vi "port_waveform_builder.vi"(4 "Line 7":digitalwaveform(waveform)={"t0"=timestamp(0 s since 1904-01-01), "dt"=0.0, "Y"={"transitions"=[], "data"=[]}, "error"={"status"=FALSE, "code"=37421928, "source"=""}}, 6 "Line 6":digitalwaveform(waveform)={"t0"=timestamp(0 s since 1904-01-01), "dt"=0.0, "Y"={"transitions"=[], "data"=[]}, "error"={"status"=FALSE, "code"=37421928, "source"=""}}, 7 "Line 1":digitalwaveform(waveform)={"t0"=timestamp(0 s since 1904-01-01), "dt"=0.0, "Y"={"transitions"=[], "data"=[]}, "error"={"status"=FALSE, "code"=37421928, "source"=""}}, 8 "Line 5":digitalwaveform(waveform)={"t0"=timestamp(0 s since 1904-01-01), "dt"=0.0, "Y"={"transitions"=[], "data"=[]}, "error"={"status"=FALSE, "code"=37421928, "source"=""}}, 11 "Line 2":digitalwaveform(waveform)={"t0"=timestamp(0 s since 1904-01-01), "dt"=0.0, "Y"={"transitions"=[], "data"=[]}, "error"={"status"=FALSE, "code"=37421928, "source"=""}}) -> (3 "digital waveform out":digitalwaveform(waveform)={"t0"=timestamp(0 s since 1904-01-01), "dt"=0.0, "Y"={"transitions"=[], "data"=[]}, "error"={"status"=FALSE, "code"=37421928, "source"=""}})   [LabVIEW 2012]
uses:
  <vilib>/Waveform/DWDTOps.llb/DWDT Append Digital Signals.vi
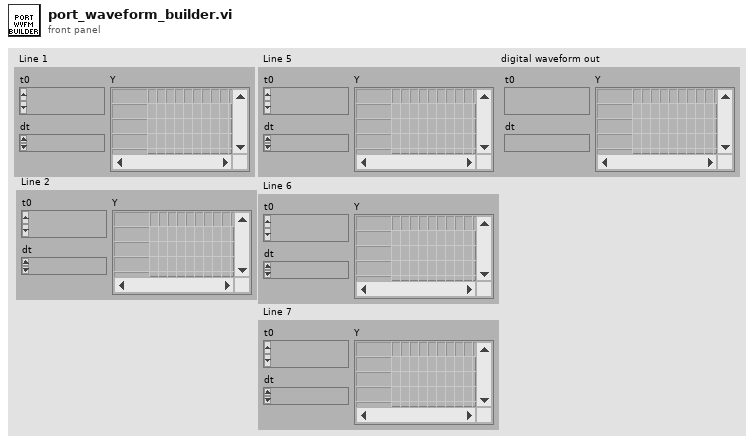
[diagram p1: front panel]
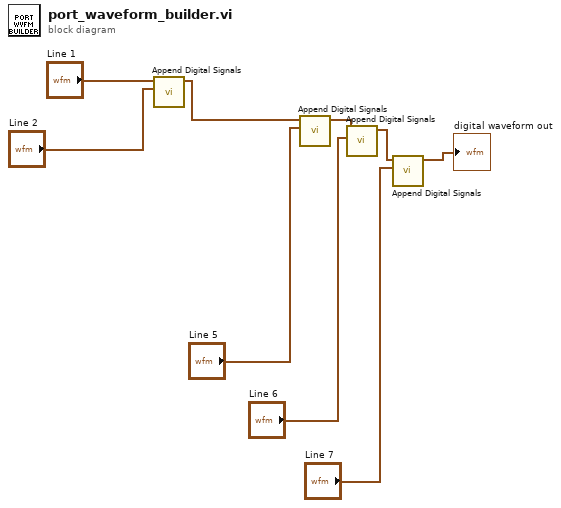
[diagram p0: block diagram]
diagram:
  n1 = call-poly <vilib>:"Append Digital Signals.vi"("digital waveform (low bits)"="Line 2", "digital waveform (high bits)"="Line 1") -> ("digital waveform out"=w1:digitalwaveform)  [unwired: 8 in, 1 out]
  n2 = call-poly <vilib>:"Append Digital Signals.vi"("digital waveform (low bits)"="Line 5", "digital waveform (high bits)"=w1) -> ("digital waveform out"=w5:digitalwaveform)  [unwired: 8 in, 1 out]
  n3 = call-poly <vilib>:"Append Digital Signals.vi"("digital waveform (low bits)"="Line 6", "digital waveform (high bits)"=w5) -> ("digital waveform out"=w6:digitalwaveform)  [unwired: 8 in, 1 out]
  n4 = call-poly <vilib>:"Append Digital Signals.vi"("digital waveform (low bits)"="Line 7", "digital waveform (high bits)"=w6) -> ("digital waveform out"=→"digital waveform out":digitalwaveform)  [unwired: 8 in, 1 out]
